vi "chart_data.vi"() -> (3 "Output Graphs":cluster{"all rows":dbl[], "all rows":dbl[]}[](array[cluster]))   [LabVIEW 2017]
panel:
  out "size(s) 5":i32
  out "size(s) 4":i32
  out "size(s) 3":i32
  out "size(s) 2":i32
  out "size(s)":i32
  out "Super_Heated_T_Curves":T1(ring)
  out "Super_Heated_S_Curves":enum16{"P", "S", "H gas"}(ring)
  out "Super_Heated_T_Curves":T2
  out "Super_Heated_S_Curves":T3
  out "Sat_Deg_10_Step":T4(ring)
  out "Sat_Deg_10_Step":T5
  out "Sat_By_Deg":T4(ring)
  out "Sat_By_Deg":T6
  out "Saturation Degrees( 10 Steps )":dbl[][](array[numeric])
  out "Sat_By_Deg_Arr":dbl[][](array[numeric])
  out "Super_Heated_S_Curves":dbl[][](array[numeric])
  out "Super_Heated_T_Curves":dbl[][](array[numeric])
  out "Temperatures In Subcooled":cluster{dbl[], dbl[]}[](array[cluster])
  out "Saturated Vapor":cluster{"all rows":dbl[], "all rows":dbl[]}
  out "Saturated Liquid":cluster{"all rows":dbl[], "all rows":dbl[]}
  out "Temperature In Super Heated":cluster{dbl[], dbl[]}[](array[cluster])
  out "S In Super heated":cluster{dbl[], dbl[]}[](array[cluster])
  out "Temperatures In Saturation":cluster{dbl[], dbl[]}[](array[cluster])
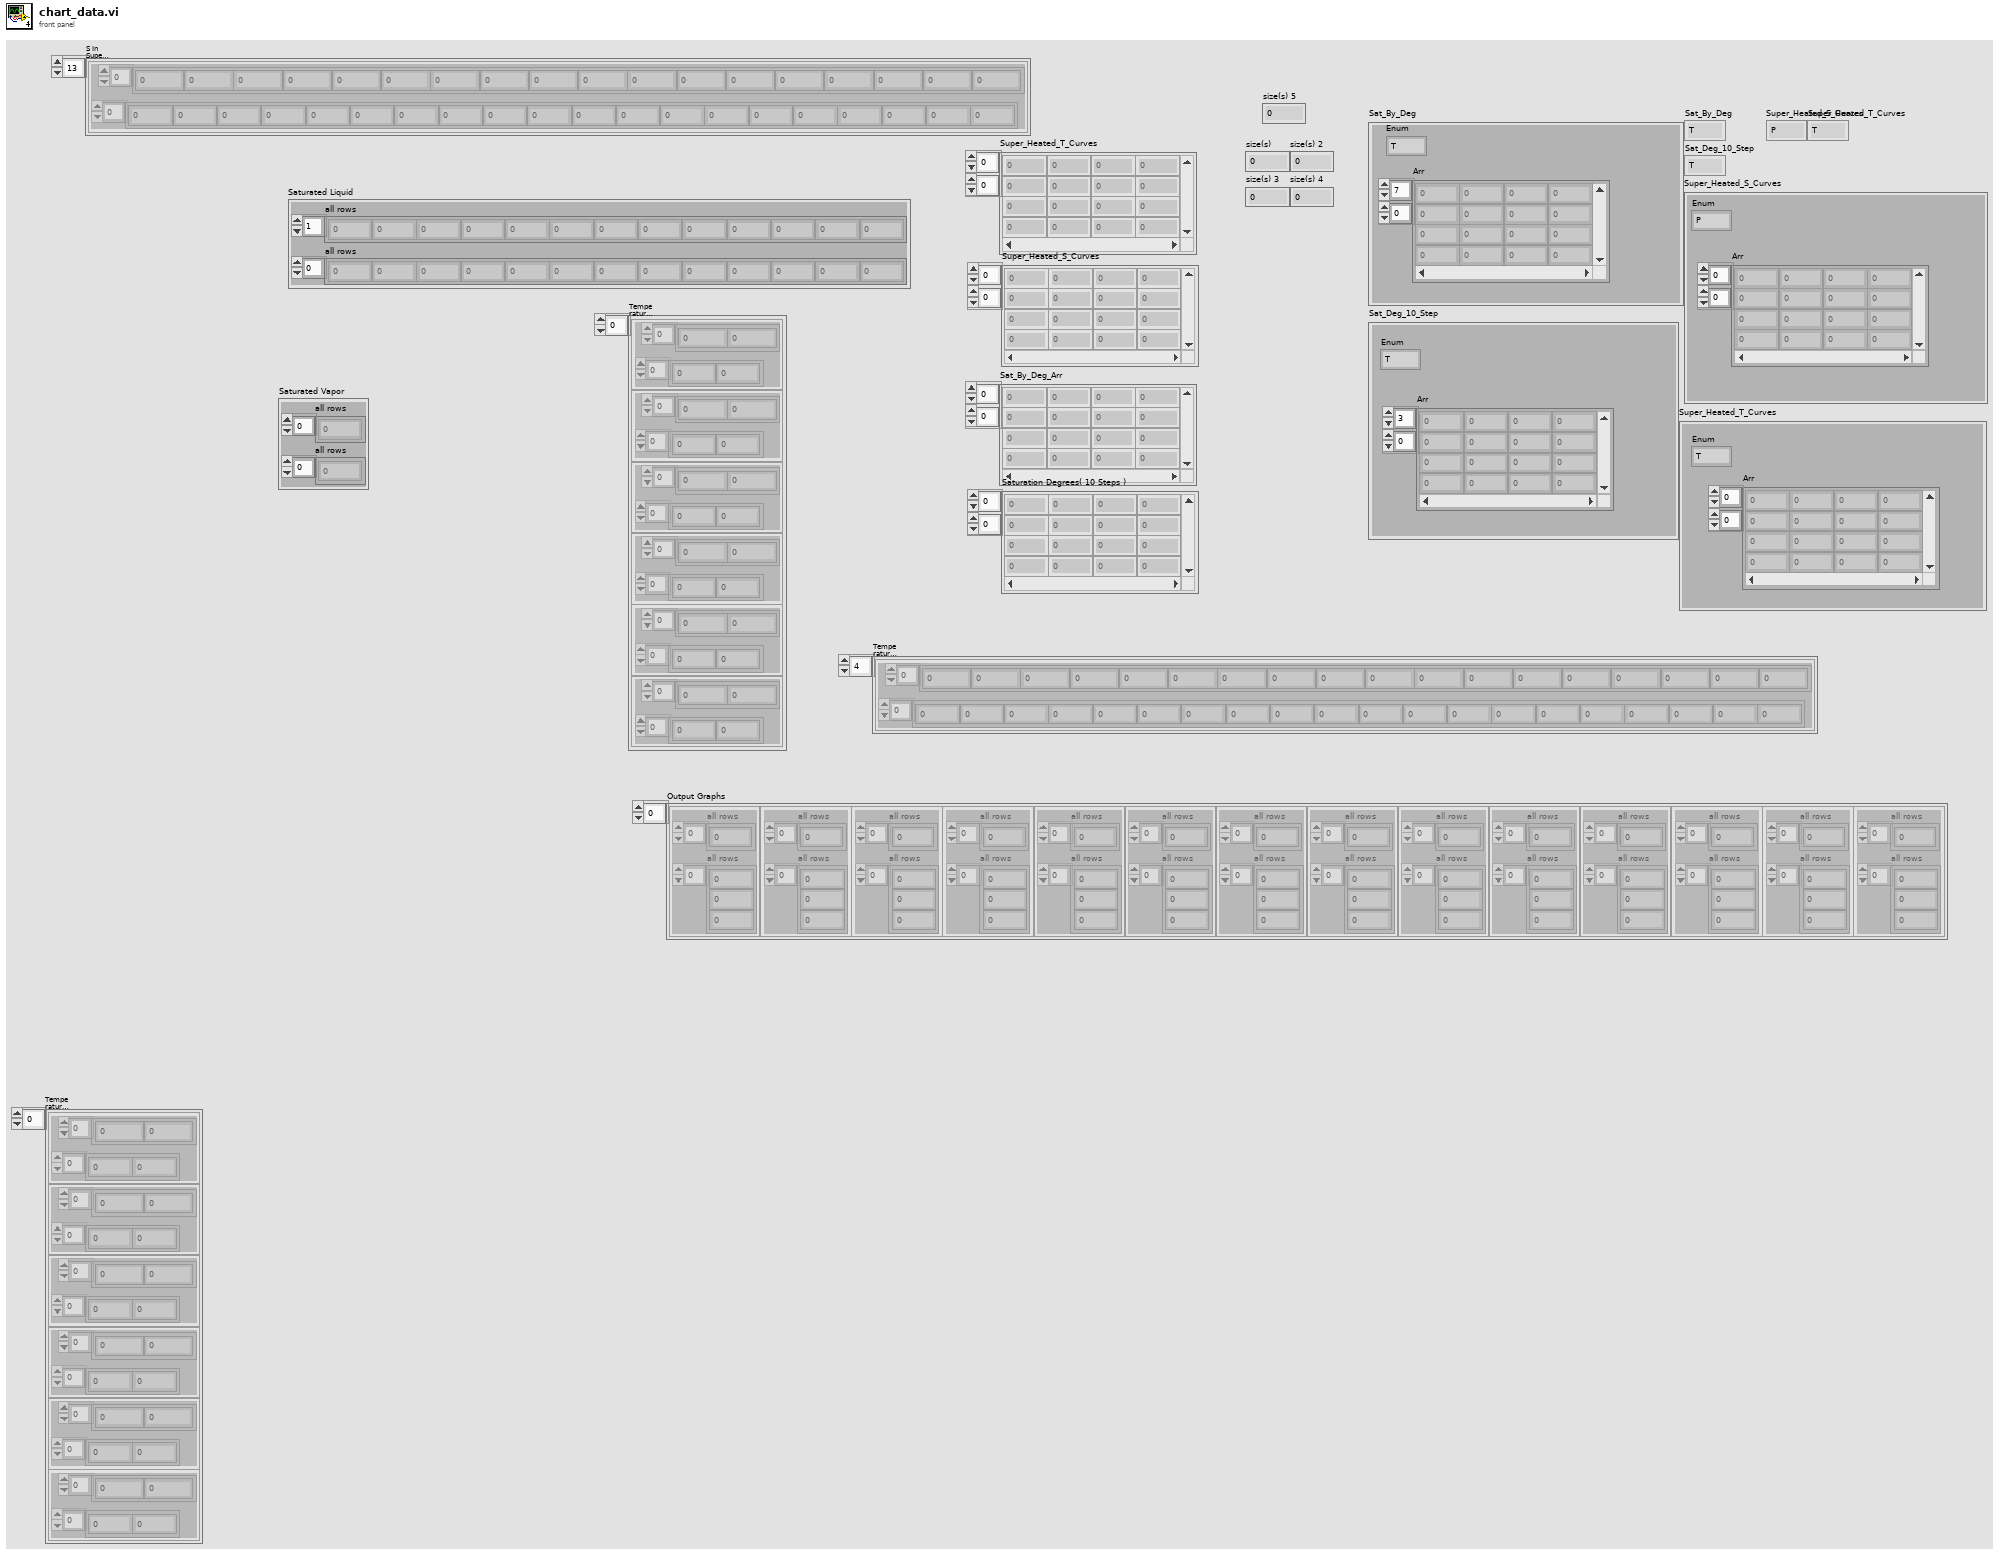
[diagram p1: front panel]
types:
  T1 = enum16{"T", "P", "T_Sat_Vapor", "Hg", "Sg", "Vg"}
  T2 = cluster{"Enum":enum16{"T", "P", "T_Sat_Vapor", "Hg", "Sg", "Vg"}, "Arr":dbl[][]}
  T3 = cluster{"Enum":enum16{"P", "S", "H gas"}, "Arr":dbl[][]}
  T4 = enum16{"T", "P", "V1", "Vg", "H1", "Hg", "R", "S1", "Sg"}
  T5 = cluster{"Enum":enum16{"T", "P", "V1", "Vg", "H1", "Hg", "R", "S1", "Sg"}, "Arr":dbl[][]}
  T6 = cluster{"Enum":enum16{"T", "P", "V1", "Vg", "H1", "Hg", "R", "S1", "Sg"}, "Arr ":dbl[][]}
  T7 = cluster{"Sat_By_Deg_Arr":dbl[], "Sat_By_Deg_Arr":dbl[]}
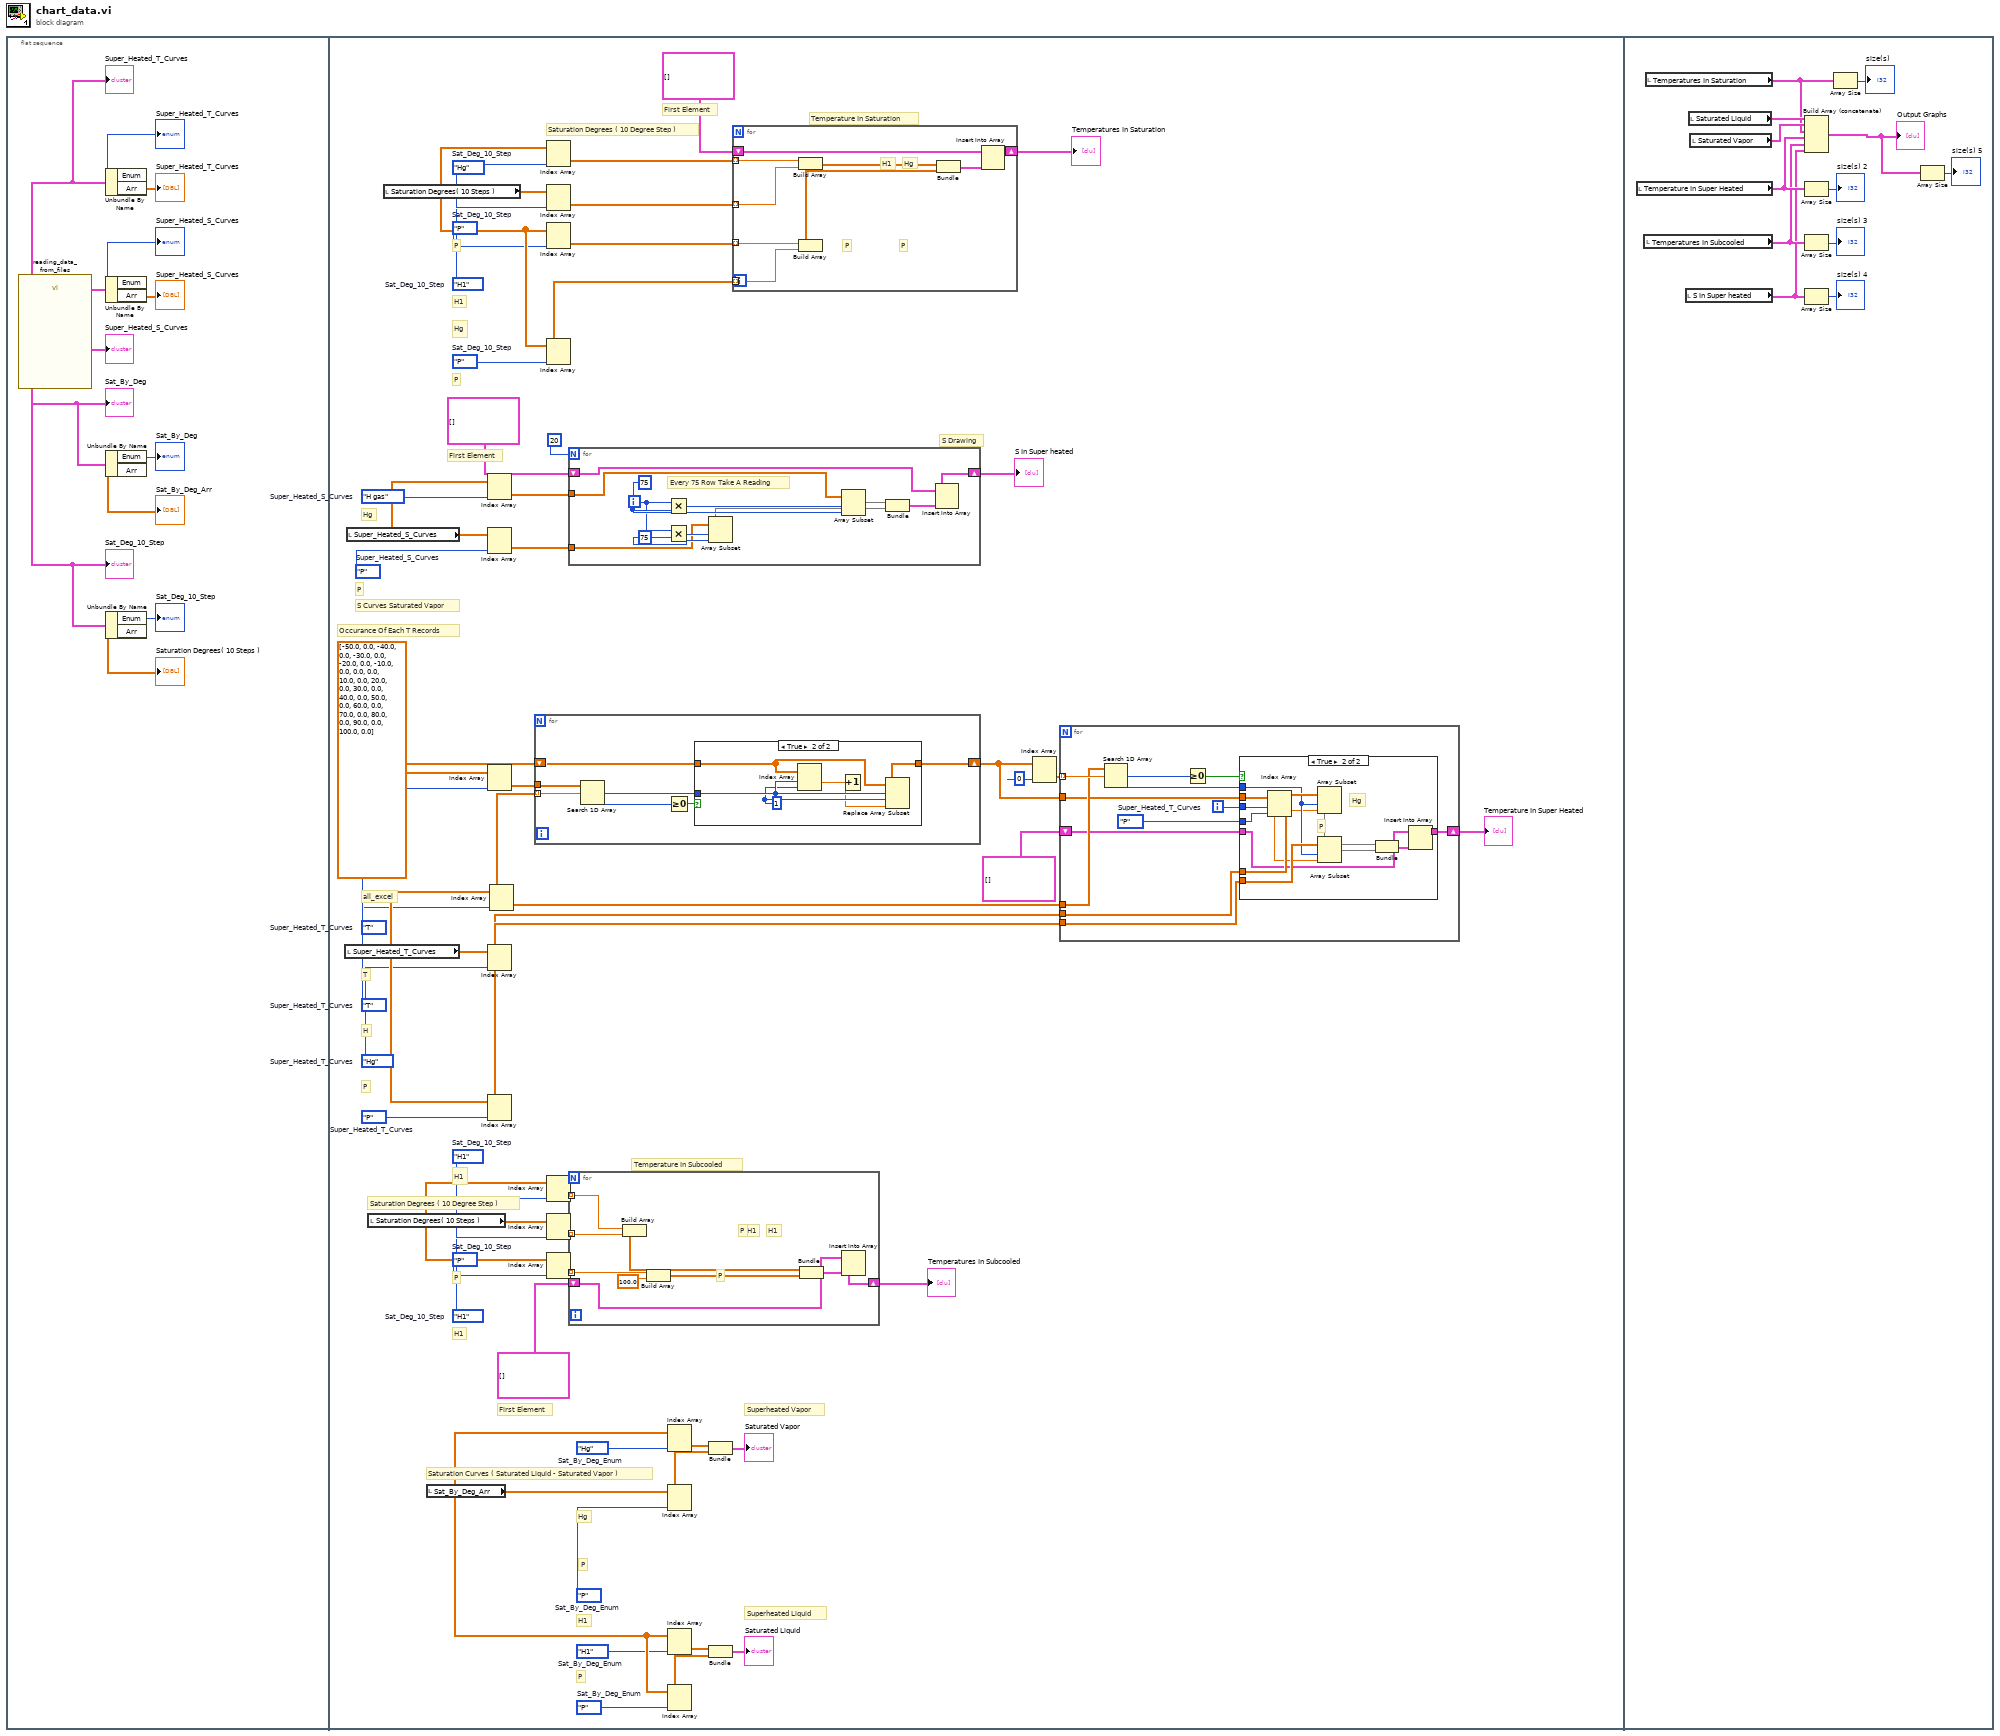
[diagram p0: block diagram]
diagram:
  n1 = flat-sequence {
    frame #0 {
      n2 = call "reading_data_from_files.vi"() -> ("Super_Heated_T_Curves"=w5:T2, "Super_Heated_S_Curves"=w6:T3, "Sat_Deg_10_Step"=w9:T5, "Sat_By_Deg"=w12:T6)  [unwired: 8 in]
      "Sat_By_Deg" <- w12
      "Sat_Deg_10_Step" <- w9
      "Super_Heated_S_Curves" <- w6
      "Super_Heated_T_Curves" <- w5
      n3 = Unbundle By Name(w5) -> ("Enum"=→"Super_Heated_T_Curves":T1, "Arr"=→"Super_Heated_T_Curves":dbl[][])
      n4 = Unbundle By Name(w6) -> ("Enum"=→"Super_Heated_S_Curves":enum16{"P", "S", "H gas"}, "Arr"=→"Super_Heated_S_Curves":dbl[][])
      n5 = Unbundle By Name(w12) -> ("Enum"=→"Sat_By_Deg":T4, "Arr"=→"Sat_By_Deg_Arr":dbl[][])
      n6 = Unbundle By Name(w9) -> ("Enum"=→"Sat_Deg_10_Step":T4, "Arr"=→"Saturation Degrees( 10 Steps )":dbl[][])
    }
    frame #1 {
      w24 = T1."P"  # Super_Heated_T_Curves
      w23 = T1."Hg"  # Super_Heated_T_Curves
      w22 = T1."T"  # Super_Heated_T_Curves
      w29 = T1."T"  # Super_Heated_T_Curves
      w28 = enum16{"P", "S", "H gas"}."P"  # Super_Heated_S_Curves
      w27 = enum16{"P", "S", "H gas"}."H gas"  # Super_Heated_S_Curves
      w36 = T4."H1"  # Sat_Deg_10_Step
      w35 = T4."P"  # Sat_Deg_10_Step
      w34 = T4."H1"  # Sat_Deg_10_Step
      w21 = T4."P"  # Sat_Deg_10_Step
      w20 = T4."Hg"  # Sat_Deg_10_Step
      w19 = T4."P"  # Sat_Deg_10_Step
      w18 = T4."H1"  # Sat_Deg_10_Step
      w16 = T4."P"  # Sat_By_Deg_Enum
      w15 = T4."Hg"  # Sat_By_Deg_Enum
      w14 = T4."P"  # Sat_By_Deg_Enum
      w13 = T4."H1"  # Sat_By_Deg_Enum
      w32 = dbl[][] [[-50.0, 0.0], [-40.0, 0.0], [-30.0, 0.0], [-20.0, 0.0], [-10.0, 0.0], [0.0, 0.0], [10.0, 0.0], [20.0, 0.0], [30.0, 0.0], [40.0, 0.0], [50.0, 0.0], [60.0, 0.0], [70.0, 0.0], [80.0, 0.0], [90.0, 0.0], [100.0, 0.0]]
      # "all_excel"
      # "Saturation Degrees ( 10 Degree Step )"
      # "Saturation Degrees ( 10 Degree Step )"
      # "Saturation Curves ( Saturated Liquid - Saturated Vapor )"
      # "H1"
      # "P"
      # "H1"
      # "First Element"
      # "Temperature In Subcooled"
      # "Occurance Of Each T Records"
      # "P"
      # "Hg"
      # "First Element"
      # "S Curves Saturated Vapor"
      # "S Drawing"
      # "P"
      # "Hg"
      # "P"
      # "H1"
      # "P"
      # "Hg"
      # "P"
      # "H1"
      # "H"
      # "P"
      # "T"
      # "First Element"
      # "Temperature In Saturation"
      # "Superheated Vapor"
      # "Superheated Liquid"
      n7 = local read "Super_Heated_T_Curves"() -> (w66:dbl[][])
      n8 = local read "Super_Heated_S_Curves"() -> (w65:dbl[][])
      n9 = local read "Saturation Degrees( 10 Steps )"() -> (w63:dbl[][])
      n10 = local read "Saturation Degrees( 10 Steps )"() -> (w62:dbl[][])
      n11 = local read "Sat_By_Deg_Arr"() -> (w64:dbl[][])
      n12 = Index Array(array=w65, index (col)=w27) -> (element=w46:dbl[])  [unwired: 1 in]
      n13 = Index Array(array=w65, index (col)=w28) -> (element=w47:dbl[])  [unwired: 1 in]
      n14 = Index Array(array=w32, index (col)=w29) -> (element=w49:dbl[])  [unwired: 1 in]
      n15 = Index Array(array=w66, index (col)=w23) -> (element=w51:dbl[])  [unwired: 1 in]
      n16 = Index Array(array=w66, index (col)=w24) -> (element=w52:dbl[])  [unwired: 1 in]
      n17 = Index Array(array=w66, index (col)=w22) -> (element=w50:dbl[])  [unwired: 1 in]
      n18 = for {
        tunnel: w50 -> [w81] mode=indexing
        tunnel: w49 -> [w80]
        shift-right: [w77] -> w54
        shift-left: w32 -> [w76]
        n19 = Search 1D Array(1D array=w80, element=w81) -> (index of element=w78:i32)  [unwired: 1 in]
        n20 = Greater Or Equal To 0?(x=w78) -> (x >= 0?=w79:bool)
        n21 = case shown="True" w79 {
          tunnel: w76 -> [w82 w88]
          tunnel: w78 -> [_ w87]
          tunnel: [w82 w83] -> w77
          frame False {
          }
          frame True {
            w85 = 1 ("disabled index (col)")
            n22 = Index Array(array=w88, index (row)=w87, index (col)=w85) -> (element=w86:dbl)
            n23 = Increment(x=w86) -> (x+1=w84:dbl)
            n24 = Replace Array Subset(array=w88, new element=w84, index (row)=w87, index (col)=w85) -> (w83:dbl[][])
          }
        }
      }
      n25 = Index Array(array=w62, index (col)=w18) -> (element=w40:dbl[])  [unwired: 1 in]
      n26 = Index Array(array=w62, index (col)=w20) -> (element=w41:dbl[])  [unwired: 1 in]
      n27 = Index Array(array=w62, index (col)=w19) -> (element=w42:dbl[])  [unwired: 1 in]
      n28 = Index Array(array=w62, index (col)=w21) -> (element=w43:dbl[])  [unwired: 1 in]
      n29 = Index Array(array=w63, index (col)=w34) -> (element=w58:dbl[])  [unwired: 1 in]
      n30 = Index Array(array=w63, index (col)=w36) -> (element=w59:dbl[])  [unwired: 1 in]
      n31 = Index Array(array=w63, index (col)=w35) -> (element=w60:dbl[])  [unwired: 1 in]
      n32 = for {
        N: 20 -> [_]
        shift-right: [w123] -> w48
        shift-left: cluster{dbl[], dbl[]}[] [] -> [w122]
        tunnel: w46 -> [w121]
        tunnel: w47 -> [w116]
        i -> [w115]
        w117 = 75 ("length")
        w119 = 75 ("length")
        # "Every 75 Row Take A Reading"
        n33 = Multiply(x=w115, y=w119) -> (x*y=w120:i32)
        n34 = Multiply(x=w115, y=w117) -> (x*y=w118:i32)
        n35 = Array Subset(array=w116, index=w118, length=w117) -> (w113:dbl[])
        n36 = Array Subset(array=w121, index=w120, length=w119) -> (w114:dbl[])
        n37 = Bundle(w114, w113) -> (w124:cluster{dbl[], dbl[]})  [unwired: 1 in]
        n38 = Insert Into Array(array=w122, new element=w124) -> (w123:cluster{dbl[], dbl[]}[])  [unwired: 1 in]
      }
      "S In Super heated" <- w48
      n39 = for {
        tunnel: w58 -> [w73] mode=indexing
        tunnel: w59 -> [w72] mode=indexing
        tunnel: w60 -> [w71] mode=indexing
        shift-right: [w68] -> w61
        shift-left: cluster{dbl[], dbl[]}[] [] -> [w69]
        # "P"
        # "P"
        # "H1"
        # "H1"
        n40 = Build Array(w73, w72) -> (w75:dbl[])
        n41 = Build Array(w71, 100.0 ("element")) -> (w74:dbl[])
        n42 = Bundle(w75, w74) -> (w70:cluster{dbl[], dbl[]})  [unwired: 1 in]
        n43 = Insert Into Array(array=w69, new element=w70) -> (w68:cluster{dbl[], dbl[]}[])  [unwired: 1 in]
      }
      "Temperatures In Subcooled" <- w61
      n44 = Index Array(array=w64, index (col)=w15) -> (element=w38:dbl[])  [unwired: 1 in]
      n45 = Index Array(array=w64, index (col)=w16) -> (element=w39:dbl[])  [unwired: 1 in]
      n46 = Index Array(array=w64, index (col)=w13) -> (element=w37:dbl[])  [unwired: 1 in]
      n47 = Index Array(array=w64, index (col)=w14) -> (element=w45:dbl[])  [unwired: 1 in]
      n48 = Bundle("Sat_By_Deg_Arr"=w38, "Sat_By_Deg_Arr"=w39) -> (→"Saturated Vapor":T7)  [unwired: 1 in]
      n49 = Bundle("Sat_By_Deg_Arr"=w37, "Sat_By_Deg_Arr"=w45) -> (→"Saturated Liquid":T7)  [unwired: 1 in]
      n50 = for {
        tunnel: w40 -> [w131] mode=indexing
        tunnel: w41 -> [w130] mode=indexing
        tunnel: w42 -> [w129] mode=indexing
        tunnel: w43 -> [w128] mode=indexing
        shift-right: [w125] -> w44
        shift-left: cluster{dbl[], dbl[]}[] [] -> [w126]
        # "P"
        # "P"
        # "Hg"
        # "H1"
        n51 = Build Array(w131, w130) -> (w133:dbl[])
        n52 = Build Array(w129, w128) -> (w132:dbl[])
        n53 = Bundle(w133, w132) -> (w127:cluster{dbl[], dbl[]})  [unwired: 1 in]
        n54 = Insert Into Array(array=w126, new element=w127) -> (w125:cluster{dbl[], dbl[]}[])  [unwired: 1 in]
      }
      "Temperatures In Saturation" <- w44
      n55 = Index Array(array=w54, index (col)=0) -> (element=w53:dbl[])  [unwired: 1 in]
      n56 = for {
        tunnel: w53 -> [w99] mode=indexing
        tunnel: w50 -> [w98]
        tunnel: w51 -> [w96]
        tunnel: w52 -> [w95]
        tunnel: w54 -> [w93]
        shift-right: [w90] -> w55
        shift-left: cluster{dbl[], dbl[]}[] [] -> [w91]
        i -> [w92]
        w89 = T1."P"  # Super_Heated_T_Curves
        n57 = Search 1D Array(1D array=w98, element=w99) -> (index of element=w94:i32)  [unwired: 1 in]
        n58 = Greater Or Equal To 0?(x=w94) -> (x >= 0?=w97:bool)
        n59 = case shown="True" w97 {
          tunnel: w96 -> [_ w112]
          tunnel: w95 -> [_ w111]
          tunnel: w94 -> [_ w110]
          tunnel: w93 -> [_ w109]
          tunnel: w92 -> [_ w108]
          tunnel: w91 -> [w100 w104]
          tunnel: [w100 w103] -> w90
          tunnel: w89 -> [_ w101]
          frame False {
          }
          frame True {
            # "P"
            # "Hg"
            n60 = Index Array(array=w109, index (row)=w108, index (col)=w101) -> (element=w107:dbl)
            n61 = Array Subset(array=w112, index=w110, length=w107) -> (w106:dbl[])
            n62 = Array Subset(array=w111, index=w110, length=w107) -> (w105:dbl[])
            n63 = Bundle(w106, w105) -> (w102:cluster{dbl[], dbl[]})  [unwired: 1 in]
            n64 = Insert Into Array(array=w104, new element=w102) -> (w103:cluster{dbl[], dbl[]}[])  [unwired: 1 in]
          }
        }
      }
      "Temperature In Super Heated" <- w55
    }
    frame #2 {
      n65 = local read "Temperature In Super Heated"() -> (w141:cluster{dbl[], dbl[]}[])
      n66 = local read "Temperatures In Subcooled"() -> (w140:cluster{dbl[], dbl[]}[])
      n67 = local read "Temperatures In Saturation"() -> (w143:cluster{dbl[], dbl[]}[])
      n68 = local read "S In Super heated"() -> (w139:cluster{dbl[], dbl[]}[])
      n69 = local read "Saturated Liquid"() -> (w145:cluster{"all rows":dbl[], "all rows":dbl[]})
      n70 = local read "Saturated Vapor"() -> (w144:cluster{"all rows":dbl[], "all rows":dbl[]})
      n71 = Build Array (concatenate)(w145, w144, w143, w141, w140, w139) -> (w135:cluster{"all rows":dbl[], "all rows":dbl[]}[])
      "Output Graphs" <- w135
      n72 = Array Size(array=w141) -> (size(s)=→"size(s) 2":i32)
      n73 = Array Size(array=w140) -> (size(s)=→"size(s) 3":i32)
      n74 = Array Size(array=w139) -> (size(s)=→"size(s) 4":i32)
      n75 = Array Size(array=w143) -> (size(s)=→"size(s)":i32)
      n76 = Array Size(array=w135) -> (size(s)=→"size(s) 5":i32)
    }
  }
